vi "Cycle Timing.vi"(8 "error in (no error)":errorcluster, 10 "iteration":i32, 11 "UI Pointers":T1) -> (0 "error out":errorcluster)   [LabVIEW 2020]
uses:
  User Interface Pointers.ctl
  <vilib>/NI/Memory Manager/Classes/Pointer/Pointer.lvclass
  <vilib>/NI/Memory Manager/Classes/Pointer/Pointer.lvclass/Pointer.ctl
  <vilib>/NI/Memory Manager/Classes/Pointer/Write I32.vi
  <vilib>/NI/Memory Manager/Classes/Pointer/Read U32.vi
  <vilib>/NI/Memory Manager/Classes/Pointer/Write U32.vi
  <vilib>/NI/Memory Manager/Classes/Pointer/Write (No Check).vi
  <vilib>/NI/Memory Manager/Classes/Pointer/Write (No Check) I32.vi
  <vilib>/NI/Memory Manager/Classes/Pointer/Check Move.vi
  <vilib>/NI/Memory Manager/Classes/Pointer/Read (No Check).vi
  <vilib>/NI/Memory Manager/Classes/Pointer/Read (No Check) U32.vi
  <vilib>/NI/Memory Manager/Classes/Pointer/Write (No Check) U32.vi
  <vilib>/NI/Memory Manager/Classes/Pointer/Get Address.vi
  <vilib>/NI/Memory Manager/Classes/Pointer/Check Null Pointer.vi
  <vilib>/NI/Memory Manager/Classes/Pointer/Check Count.vi
  <vilib>/NI/Memory Manager/Classes/Pointer/Check Bounds (Power of 2).vi
  <vilib>/NI/Memory Manager/Classes/Pointer/Errors.vi
  <vilib>/NI/Memory Manager/Classes/Pointer/Null Pointer.vi
  <vilib>/NI/Memory Manager/Classes/Pointer/Is Null.vi
  <vilib>/NI/Memory Manager/Classes/Pointer/Get Size.vi
  <vilib>/NI/Memory Manager/Classes/Pointer/Out of Bounds.vi
  <vilib>/NI/Memory Manager/Classes/Pointer/Check Bounds.vi
  <vilib>/NI/Memory Manager/Classes/Pointer/Create Error.vi
  <vilib>/NI/Memory Manager/VIs/Write String to Source.vi
  <vilib>/NI/Memory Manager/Classes/Pointer/Write Pointer Size to Error.vi
  <vilib>/NI/Memory Manager/VIs/Write Numeric to Source.vi
  <vilib>/NI/Memory Manager/VIs/Write Numeric Scalar to Source (Base10 U64).vi
  <vilib>/NI/Memory Manager/Classes/Pointer/Check Bounds (Pointer).vi
  <vilib>/NI/Memory Manager/Classes/Pointer/Check Bounds (Buffer).vi
  <vilib>/NI/Memory Manager/VIs/New Error Cluster.vi
  <vilib>/NI/Memory Manager/VIs/New Error Cluster (512B).vi
  <vilib>/NI/Memory Manager/VIs/Set Error Status.vi
  <vilib>/NI/Memory Manager/VIs/Set Error Code.vi
  <vilib>/NI/Memory Manager/VIs/Set Error Source.vi
  <vilib>/NI/Memory Manager/Constants/Constants.vi
  <vilib>/NI/Memory Manager/Constants/Library Name.vi
  <vilib>/NI/Memory Manager/Classes/Pointer/Pointer Error Info.vi
  <vilib>/NI/Memory Manager/Constants/Pointer Class Name.vi
  <vilib>/NI/Memory Manager/Classes/Pointer/Buffer Underflow.vi
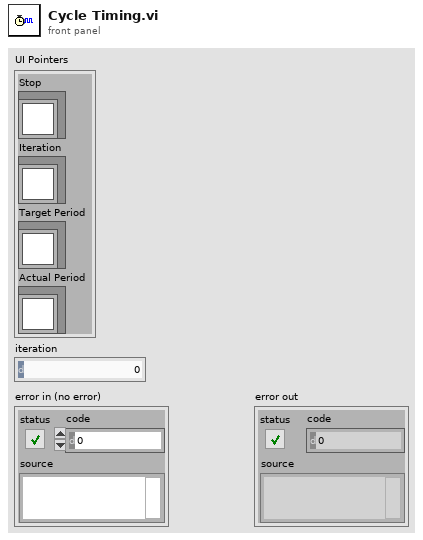
[diagram p1: front panel]
types:
  T1 = typedef "User Interface Pointers.ctl" = cluster{"Stop":refnum<class "Pointer.lvclass">, "Iteration":refnum<class "Pointer.lvclass">, "Target Period":refnum<class "Pointer.lvclass">, "Actual Period":refnum<class "Pointer.lvclass">}
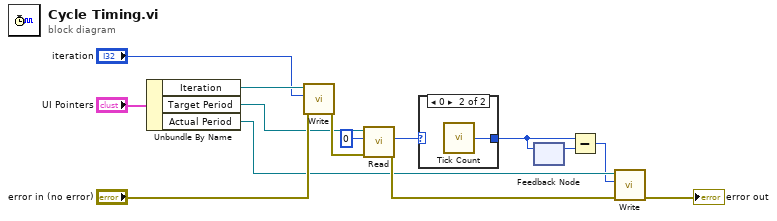
[diagram p0: block diagram]
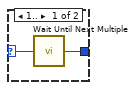
[diagram p2: hidden frame]
diagram:
  n1 = Unbundle By Name("UI Pointers") -> ("Iteration"=w7:refnum<class "Pointer.lvclass">, "Target Period"=w3:refnum<class "Pointer.lvclass">, "Actual Period"=w2:refnum<class "Pointer.lvclass">)
  n2 = call-poly <vilib>:"Write.vi"("error in (no error)"="error in (no error)", "value"="iteration", "Pointer in"=w7) -> ("error out"=w12:errorcluster)  [unwired: 5 in, 3 out]
  n3 = call-poly <vilib>:"Read.vi"("error in (no error)"=w12, "value in"=u32 0, "Pointer in"=w3) -> ("error out"=w13:errorcluster, "value out"=w10:u32)  [unwired: 5 in, 2 out]
  n4 = case shown="0" w10 {
    selector: w10 -> [w15 _]
    tunnel: [w16 w17] -> w11
    frame 1.. {
      n5 = call "Wait Until Next Multiple"("Count(uSec)"=w15) -> ("Tick Count(uSec)"=w16:u32)
    }
    frame 0 {
      n6 = call "Tick Count"() -> ("Tick Count(uSec)"=w17:u32)
    }
  }
  n7 = feedback #1() -> (w14:u32)  [unwired: 1 in]
  n8 = feedback-in #1(w11) -> ()
  n9 = Subtract(x=w11, y=w14) -> (x-y=w1:u32)
  n10 = call-poly <vilib>:"Write.vi"("error in (no error)"=w13, "value"=w1, "Pointer in"=w2) -> ("error out"=→"error out":errorcluster)  [unwired: 5 in, 3 out]
